vi "Parse String.vi"(11 "Pattern String":string) -> (3 "Pattern":T1)   [LabVIEW 2020, in "Stream.lvlib" / "URLPattern.lvclass"]
uses:
  URLPattern.lvclass
  URL Pattern Init.ctl
panel:
  out "x >= 0?":bool
  out "Scheme After":string
  out "Scheme Before":string
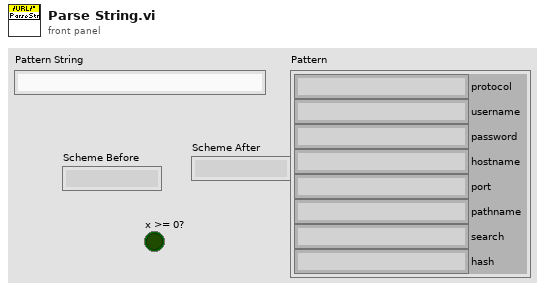
[diagram p1: front panel]
types:
  T1 = typedef "Stream.lvlib/URLPattern.lvclass/URL Pattern Init.ctl" = cluster{"protocol":string, "username":string, "password":string, "hostname":string, "port":string, "pathname":string, "search":string, "hash":string}
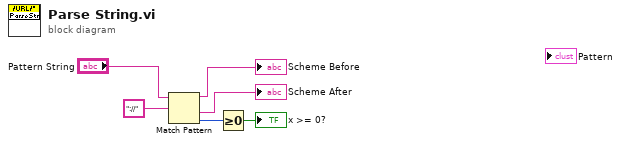
[diagram p0: block diagram]
diagram:
  n1 = Match Pattern(string="Pattern String", regular expression="://") -> (before substring=→"Scheme Before":string, after substring=→"Scheme After":string, offset past match=w2:i32)  [unwired: 1 in, 1 out]
  n2 = Greater Or Equal To 0?(x=w2) -> (x >= 0?=→"x >= 0?":bool)
